vi "Update Controller State.vi"(8 "error in (no error)":errorcluster, 11 "Elevator Controller in":refnum<class "Elevator Controller.lvclass">) -> (0 "error out":errorcluster, 3 "Elevator Controller out":refnum<class "Elevator Controller.lvclass">)   [LabVIEW 2019, in "Elevator Controller.lvlib" / "Elevator Controller.lvclass"]
uses:
  Elevator Controller.lvclass
  C:/Program Files (x86)/National Instruments/LabVIEW 2019/vi.lib/ActorFramework/Actor/Actor.lvclass
  <vilib>/ActorFramework/Actor/Actor.lvclass/Actor.ctl
  <vilib>/ActorFramework/Message Enqueuer/Message Enqueuer.lvclass/Message Enqueuer.ctl
  Elevator Controller.lvclass/Elevator Controller.ctl
  Sim User Console Actor/Elevator Controller/Doors -Button.ctl
  Sim User Console Actor/Elevator Controller/Elevator Call -Cluster.ctl
  Sim User Console Actor/Elevator Controller/Floor Selection -Cluster.ctl
  Sim Display Console Actor/Elevator Controller/Elevator Direction.ctl
  Sim Display Console Actor/Elevator Controller/Floors -Enum.ctl
  Configuration Database Actor/Configuration Database Actor Messages/Write DB Msg/Write DB Msg.lvclass/Write DB Msg.ctl
  Sim Sensor Interface Actor/Sim Sensor Interface Actor Messages/Write Elevator Position Msg/Write Elevator Position Msg.lvclass/Write Elevator Position Msg.ctl
  Sim Display Console Actor/Sim Display Console Actor Messages/Write Door Open Msg/Write Door Open Msg.lvclass/Write Door Open Msg.ctl
  Sim Display Console Actor/Sim Display Console Actor Messages/Write Elevator Direction Msg/Write Elevator Direction Msg.lvclass/Write Elevator Direction Msg.ctl
  Sim Display Console Actor/Sim Display Console Actor Messages/Write Elevator Location Msg/Write Elevator Location Msg.lvclass/Write Elevator Location Msg.ctl
  Sim Display Console Actor/Sim Display Console Actor Messages/Write Emergency Msg/Write Emergency Msg.lvclass/Write Emergency Msg.ctl
  Sim Display Console Actor/Sim Display Console Actor Messages/Write Timing Msg/Write Timing Msg.lvclass/Write Timing Msg.ctl
  Sim User Console Actor/Sim User Console Actor Messages/Write Doors Msg/Write Doors Msg.lvclass/Write Doors Msg.ctl
  Sim User Console Actor/Sim User Console Actor Messages/Write Elevator Call Msg/Write Elevator Call Msg.lvclass/Write Elevator Call Msg.ctl
  Sim User Console Actor/Sim User Console Actor Messages/Write Emergency Msg/Write Emergency Msg.lvclass/Write Emergency Msg.ctl
  Sim User Console Actor/Sim User Console Actor Messages/Write Floor Selection Msg/Write Floor Selection Msg.lvclass/Write Floor Selection Msg.ctl
  State -Enum.ctl
  Elevator Controller Messages/Set State Msg/Set State Msg.lvclass/Set State Msg.ctl
  Sim User Console Actor/Sim User Console Actor Messages/Enable Doors Msg/Enable Doors Msg.lvclass/Enable Doors Msg.ctl
  Sim Display Console Actor/Sim Display Console Actor Messages/Enable Open Door Msg/Enable Open Door Msg.lvclass/Enable Open Door Msg.ctl
  Sim User Console Actor/Sim User Console Actor Messages/Enable all Controls Msg/Enable all Controls Msg.lvclass/Enable all Controls Msg.ctl
  <vilib>/ActorFramework/Message Enqueuer/Init from Existing Queue.vi
  <vilib>/ActorFramework/Message Enqueuer/Enqueue.vi
  Configuration Database Actor/Configuration Database Actor Messages/Write DB Msg/Write DB Msg.lvclass
  C:/Program Files (x86)/National Instruments/LabVIEW 2019/vi.lib/ActorFramework/Message/Message.lvclass
  Configuration Database Actor/Configuration Database Actor Messages/Read DB Msg/Read DB Msg.lvclass
  Sim Sensor Interface Actor/Sim Sensor Interface Actor Messages/Write Elevator Position Msg/Write Elevator Position Msg.lvclass
  Sim Display Console Actor/Sim Display Console Actor Messages/Write Door Open Msg/Write Door Open Msg.lvclass
  Sim Display Console Actor/Sim Display Console Actor Messages/Write Elevator Direction Msg/Write Elevator Direction Msg.lvclass
  Sim Display Console Actor/Sim Display Console Actor Messages/Write Elevator Location Msg/Write Elevator Location Msg.lvclass
  Sim Display Console Actor/Sim Display Console Actor Messages/Write Emergency Msg/Write Emergency Msg.lvclass
  Sim Display Console Actor/Sim Display Console Actor Messages/Write Timing Msg/Write Timing Msg.lvclass
  Sim User Console Actor/Sim User Console Actor Messages/Write Doors Msg/Write Doors Msg.lvclass
  Sim User Console Actor/Sim User Console Actor Messages/Write Elevator Call Msg/Write Elevator Call Msg.lvclass
  Sim User Console Actor/Sim User Console Actor Messages/Write Emergency Msg/Write Emergency Msg.lvclass
  Sim User Console Actor/Sim User Console Actor Messages/Write Floor Selection Msg/Write Floor Selection Msg.lvclass
  Elevator Controller Messages/Set State Msg/Set State Msg.lvclass
  Sim User Console Actor/Sim User Console Actor Messages/Enable Doors Msg/Enable Doors Msg.lvclass
  Sim Display Console Actor/Sim Display Console Actor Messages/Read Elevator Direction Msg/Read Elevator Direction Msg.lvclass
  Sim User Console Actor/Sim User Console Actor Messages/Read All Controls Msg/Read All Controls Msg.lvclass
  Elevator Controller Messages/Analysis Msg/Analysis Msg.lvclass
  Sim Display Console Actor/Sim Display Console Actor Messages/Enable Open Door Msg/Enable Open Door Msg.lvclass
  Sim User Console Actor/Sim User Console Actor Messages/Enable all Controls Msg/Enable all Controls Msg.lvclass
  <vilib>/ActorFramework/Message Priority Queue/Priority Enqueue.vi
  <vilib>/ActorFramework/Message Enqueuer/Message Enqueuer.lvclass
  <vilib>/ActorFramework/Actor/Actor.lvclass
  Sim User Console Actor/Elevator Controller/Sim User Console Actor.lvclass
  Sim Display Console Actor/Elevator Controller/Sim Display Console Actor.lvclass
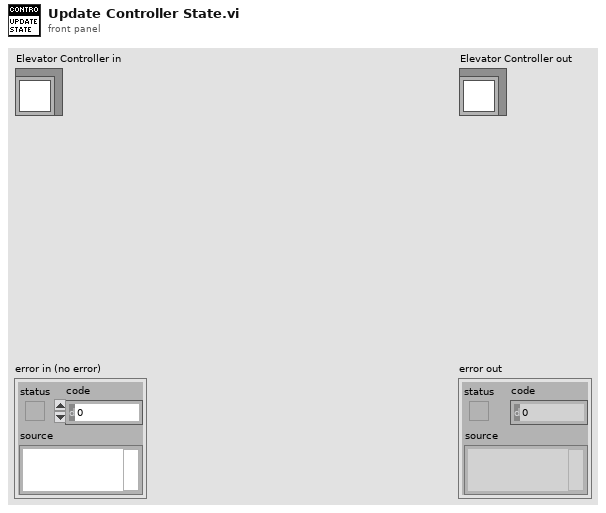
[diagram p1: front panel]
types:
  T1 = typedef "Sim Display Console Actor.lvlib/Sim Display Console Actor.lvclass/Floors -Enum.ctl" = enum16{"1st Floor", "2nd Floor", "3rd Floor", "4th Floor"}
  T2 = typedef "Sim Display Console Actor.lvlib/Sim Display Console Actor.lvclass/Elevator Direction.ctl" = cluster{"Open Door":bool, "Close Door":bool}
  T3 = typedef "Sim User Console Actor.lvlib/Sim User Console Actor.lvclass/Floor Selection -Cluster.ctl" = cluster{"4":bool, "3":bool, "2":bool, "1":bool}
  T4 = typedef "Sim User Console Actor.lvlib/Sim User Console Actor.lvclass/Elevator Call -Cluster.ctl" = cluster{"Up 3":bool, "Up 2":bool, "Up 1":bool, "Down 4":bool, "Down 3":bool, "Down 2":bool}
  T5 = typedef "Sim User Console Actor.lvlib/Sim User Console Actor.lvclass/Doors -Button.ctl" = cluster{"Open Door":bool, "Close Door":bool}
  T6 = typedef "Elevator Controller.lvlib/Elevator Controller.lvclass/State -Enum.ctl" = enum16{"Initial", "Wait for First Request", "Start and Move", "Analysis", "Continue Travel", "Stop at Floor", "Open and Close Door Sequence", "No request Remaining", "Emergency Call", "Terminate Process"}
  T7 = enum8{"Enabled", "Disabled", "Disabled and Grayed Out"}
  T8 = typedef "Configuration Database Actor.lvlib/Configuration Database Actor.lvclass/Record Data -Cluster.ctl" = cluster{"Door Open":dbl, "Door Close":dbl, "Travel Time":dbl, "Inactivity Time":dbl}
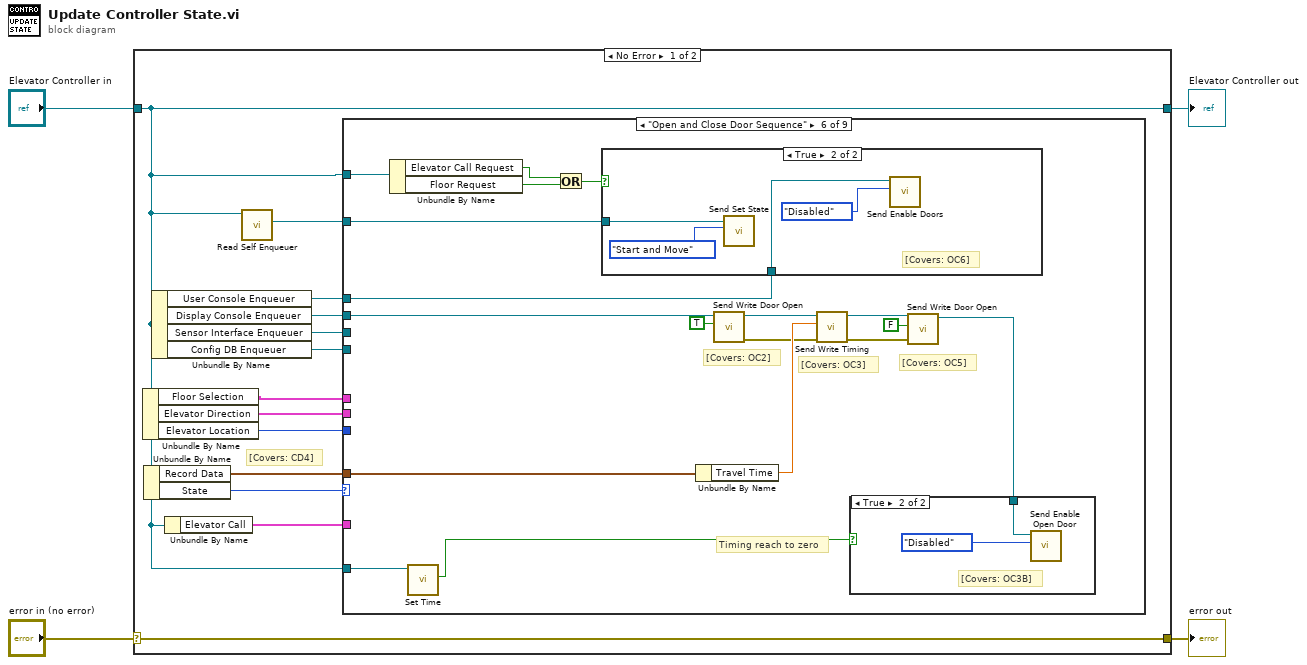
[diagram p0: block diagram]
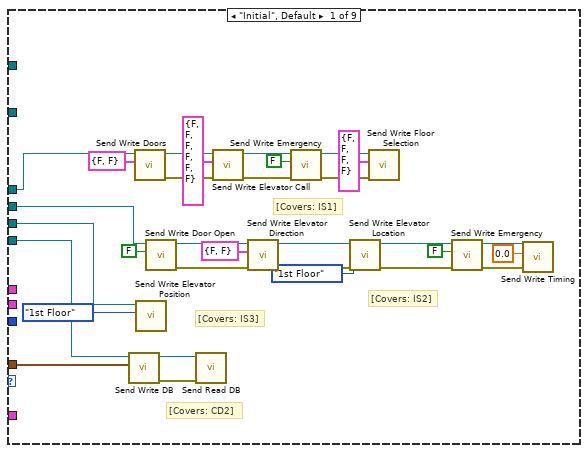
[diagram p2: hidden frame]
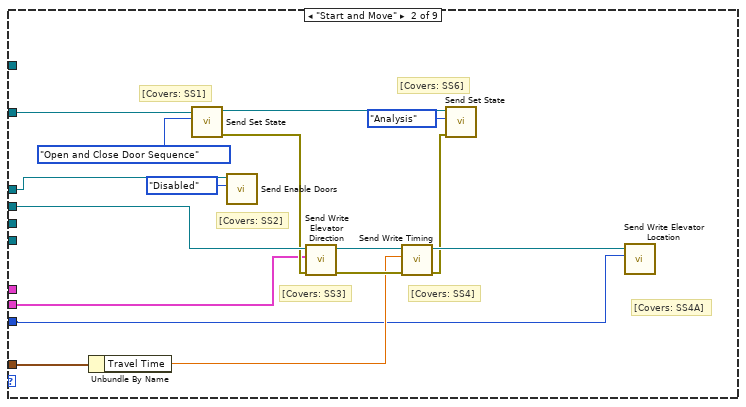
[diagram p3: hidden frame]
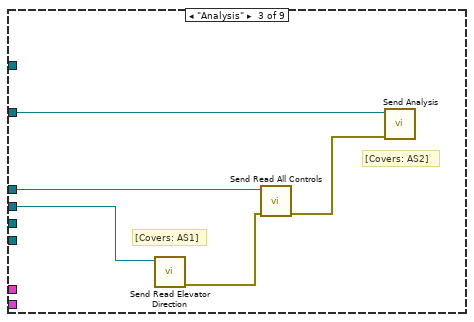
[diagram p4: hidden frame]
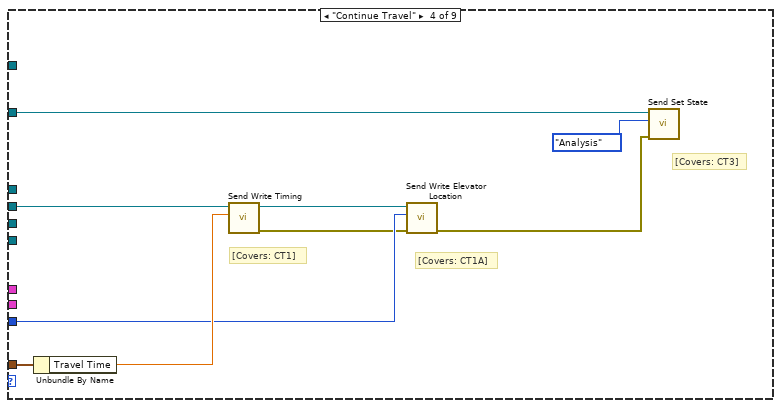
[diagram p5: hidden frame]
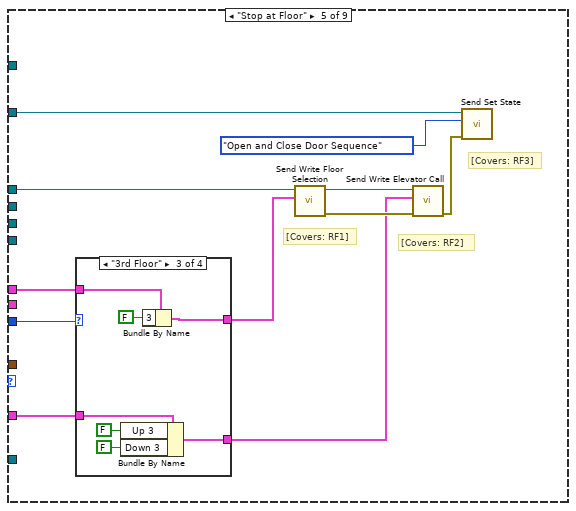
[diagram p6: hidden frame]
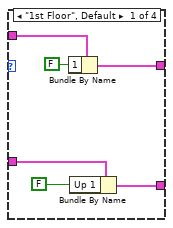
[diagram p7: hidden frame]
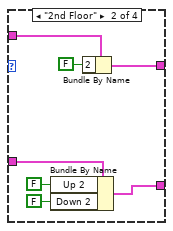
[diagram p8: hidden frame]
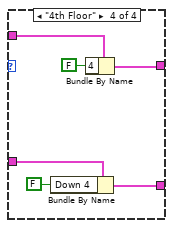
[diagram p9: hidden frame]
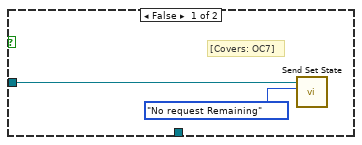
[diagram p11: hidden frame]
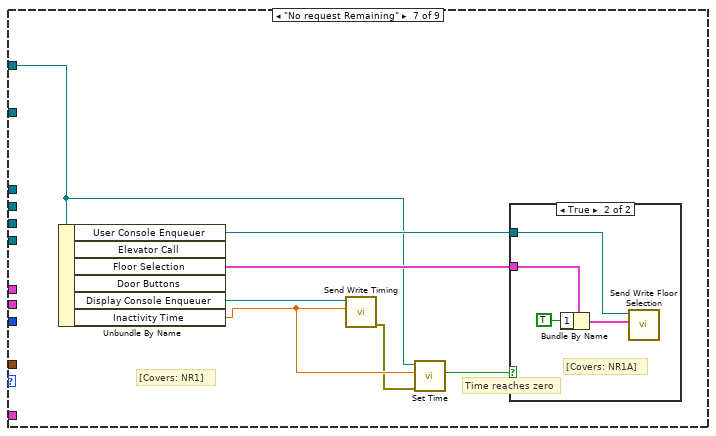
[diagram p12: hidden frame]
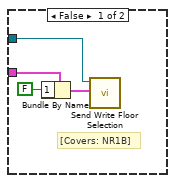
[diagram p13: hidden frame]
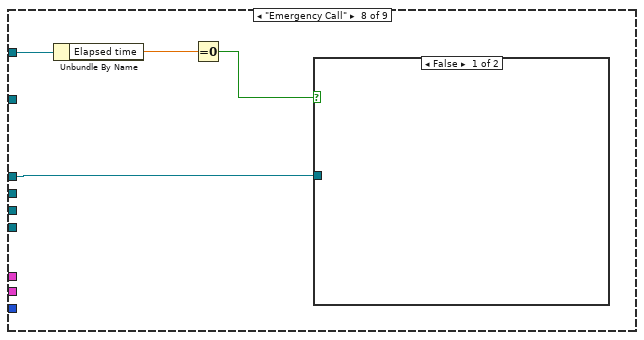
[diagram p14: hidden frame]
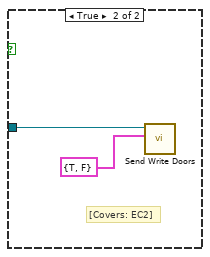
[diagram p15: hidden frame]
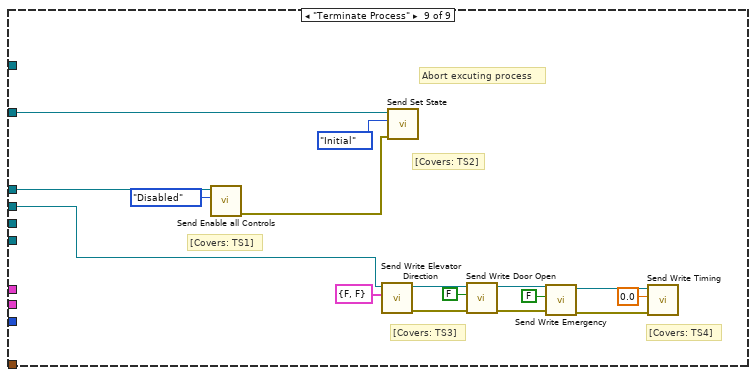
[diagram p16: hidden frame]
diagram:
  n1 = case shown="No Error" "error in (no error)" {
    selector: "error in (no error)" -> [w17 w180]
    tunnel: [w17 w180] -> w3
    tunnel: [w5 w179] -> w1
    tunnel: "Elevator Controller in" -> [w5 w179]
    frame No Error {
      # "[Covers: CD4]"
      n2 = Unbundle By Name(w5) -> ("Floor Selection"=w7:T3, "Elevator Direction"=w9:T2, "Elevator Location"=w8:T1)
      n3 = Unbundle By Name(w5) -> ("Record Data"=w10:T8, "State"=w16:T6)
      n4 = Unbundle By Name(w5) -> ("User Console Enqueuer"=w15:refnum<class "Message Enqueuer.lvclass">, "Display Console Enqueuer"=w14:refnum<class "Message Enqueuer.lvclass">, "Sensor Interface Enqueuer"=w13:refnum<class "Message Enqueuer.lvclass">, "Config DB Enqueuer"=w12:refnum<class "Message Enqueuer.lvclass">)
      n5 = Unbundle By Name(w5) -> ("Elevator Call"=w6:T4)
      n6 = call <vilib>:"Read Self Enqueuer.vi"("Actor"=w5) -> ("Self Enqueuer"=w11:refnum<class "Message Enqueuer.lvclass">)  [unwired: 10 in]
      n7 = case shown="\"Open and Close Door Sequence\"" w16 {
        tunnel: w15 -> [w44 w62 w69 _ w89 w122 _ w158 w178]
        tunnel: w14 -> [w25 w60 w68 w75 _ w133 _ _ w166]
        tunnel: w13 -> [w19 _ _ _ _ _ _ _ _]
        tunnel: w12 -> [w48 _ _ _ _ _ _ _ _]
        tunnel: w11 -> [_ w64 w67 w78 w81 w120 _ _ w176]
        tunnel: w10 -> [w45 w59 _ w76 _ w130 _ _ _]
        tunnel: w9 -> [_ w49 _ _ _ _ _ _ _]
        tunnel: w5 -> [_ _ _ _ _ w125 w142 w160 _]
        tunnel: w8 -> [_ w54 _ w72 w88 _ _ _ _]
        tunnel: w7 -> [_ _ _ _ w86 _ _ _ _]
        tunnel: w6 -> [_ _ _ _ w83 _ _ _ _]
        tunnel: w5 -> [_ _ _ _ _ w119 _ _ _]
        frame "Initial", Default {
          # "[Covers: IS3]"
          # "[Covers: IS2]"
          # "[Covers: IS1]"
          # "[Covers: CD2]"
          n8 = call "Send Write DB.vi"("Record Data"=w45, "Message Enqueuer"=w48) -> ("error out"=w46:errorcluster, "Message Enqueuer out"=w47:refnum<class "Message Enqueuer.lvclass">)  [unwired: 8 in]
          n9 = call "Send Write Doors.vi"("Door Buttons"=T5 {"Open Door"=FALSE, "Close Door"=FALSE}, "Message Enqueuer"=w44) -> ("error out"=w40:errorcluster, "Message Enqueuer out"=w43:refnum<class "Message Enqueuer.lvclass">)  [unwired: 8 in]
          n10 = call "Send Write Elevator Position.vi"("Elevator Position"=Floors_-Enum."1st Floor" ("Elevator Location"), "Message Enqueuer"=w19) -> ()  [unwired: 8 in, 2 out]
          n11 = call "Send Write Door Open.vi"("Door Open"=FALSE, "Message Enqueuer"=w25) -> ("error out"=w29:errorcluster, "Message Enqueuer out"=w33:refnum<class "Message Enqueuer.lvclass">)  [unwired: 8 in]
          n12 = call "Send Read DB.vi"("error in (no error)"=w46, "Message Enqueuer"=w47) -> ()  [unwired: 8 in, 2 out]
          n13 = call "Send Write Elevator Call.vi"("error in (no error)"=w40, "Elevator Call"=T4 {"Up 3"=FALSE, "Up 2"=FALSE, "Up 1"=FALSE, "Down 4"=FALSE, "Down 3"=FALSE, "Down 2"=FALSE}, "Message Enqueuer"=w43) -> ("error out"=w39:errorcluster, "Message Enqueuer out"=w42:refnum<class "Message Enqueuer.lvclass">)  [unwired: 7 in]
          n14 = call "Send Write Elevator Direction.vi"("error in (no error)"=w29, "Elevator Direction"=T2 {"Open Door"=FALSE, "Close Door"=FALSE}, "Message Enqueuer"=w33) -> ("error out"=w28:errorcluster, "Message Enqueuer out"=w32:refnum<class "Message Enqueuer.lvclass">)  [unwired: 7 in]
          n15 = call "Send Write Emergency.vi"("error in (no error)"=w39, "Emergency"=FALSE, "Message Enqueuer"=w42) -> ("error out"=w38:errorcluster, "Message Enqueuer out"=w41:refnum<class "Message Enqueuer.lvclass">)  [unwired: 7 in]
          n16 = call "Send Write Elevator Location.vi"("error in (no error)"=w28, "Elevator Location"=Floors_-Enum."1st Floor", "Message Enqueuer"=w32) -> ("error out"=w27:errorcluster, "Message Enqueuer out"=w31:refnum<class "Message Enqueuer.lvclass">)  [unwired: 7 in]
          n17 = call "Send Write Floor Selection.vi"("error in (no error)"=w38, "Floor Selection"=T3 {"4"=FALSE, "3"=FALSE, "2"=FALSE, "1"=FALSE}, "Message Enqueuer"=w41) -> ()  [unwired: 7 in, 2 out]
          n18 = call "Send Write Emergency.vi"("error in (no error)"=w27, "Emergency"=FALSE, "Message Enqueuer"=w31) -> ("error out"=w26:errorcluster, "Message Enqueuer out"=w30:refnum<class "Message Enqueuer.lvclass">)  [unwired: 7 in]
          n19 = call "Send Write Timing.vi"("error in (no error)"=w26, "timing"=0.0, "Message Enqueuer"=w30) -> ()  [unwired: 7 in, 2 out]
        }
        frame "Start and Move" {
          # "[Covers: SS4A]"
          # "[Covers: SS6]"
          # "[Covers: SS4]"
          # "[Covers: SS3]"
          # "[Covers: SS2]"
          # "[Covers: SS1]"
          n20 = Unbundle By Name(w59) -> ("Travel Time"=w56:dbl)
          n21 = call "Send Set State.vi"("State"=State_-Enum."Open and Close Door Sequence", "Message Enqueuer"=w64) -> ("error out"=w52:errorcluster, "Message Enqueuer out"=w51:refnum<class "Message Enqueuer.lvclass">)  [unwired: 8 in]
          n22 = call "Send Enable Doors.vi"("Disabled"=T7."Disabled", "Message Enqueuer"=w62) -> ()  [unwired: 8 in, 2 out]
          n23 = call "Send Write Elevator Direction.vi"("error in (no error)"=w52, "Elevator Direction"=w49, "Message Enqueuer"=w60) -> ("error out"=w57:errorcluster, "Message Enqueuer out"=w58:refnum<class "Message Enqueuer.lvclass">)  [unwired: 7 in]
          n24 = call "Send Write Timing.vi"("error in (no error)"=w57, "timing"=w56, "Message Enqueuer"=w58) -> ("error out"=w53:errorcluster, "Message Enqueuer out"=w55:refnum<class "Message Enqueuer.lvclass">)  [unwired: 7 in]
          n25 = call "Send Set State.vi"("error in (no error)"=w53, "State"=State_-Enum."Analysis", "Message Enqueuer"=w51) -> ()  [unwired: 7 in, 2 out]
          n26 = call "Send Write Elevator Location.vi"("Elevator Location"=w54, "Message Enqueuer"=w55) -> ()  [unwired: 8 in, 2 out]
        }
        frame "Analysis" {
          # "[Covers: AS2]"
          # "[Covers: AS1]"
          n27 = call "Send Read Elevator Direction.vi"("Message Enqueuer"=w68) -> ("error out"=w66:errorcluster)  [unwired: 9 in, 1 out]
          n28 = call "Send Read All Controls.vi"("error in (no error)"=w66, "Message Enqueuer"=w69) -> ("error out"=w65:errorcluster)  [unwired: 8 in, 1 out]
          n29 = call "Send Analysis.vi"("error in (no error)"=w65, "Message Enqueuer"=w67) -> ()  [unwired: 8 in, 2 out]
        }
        frame "Continue Travel" {
          # "[Covers: CT1A]"
          # "[Covers: CT1]"
          # "[Covers: CT3]"
          n30 = Unbundle By Name(w76) -> ("Travel Time"=w74:dbl)
          n31 = call "Send Write Timing.vi"("timing"=w74, "Message Enqueuer"=w75) -> ("error out"=w71:errorcluster, "Message Enqueuer out"=w73:refnum<class "Message Enqueuer.lvclass">)  [unwired: 8 in]
          n32 = call "Send Write Elevator Location.vi"("error in (no error)"=w71, "Elevator Location"=w72, "Message Enqueuer"=w73) -> ("error out"=w70:errorcluster)  [unwired: 7 in, 1 out]
          n33 = call "Send Set State.vi"("error in (no error)"=w70, "State"=State_-Enum."Analysis", "Message Enqueuer"=w78) -> ()  [unwired: 7 in, 2 out]
        }
        frame "Stop at Floor" {
          # "[Covers: RF3]"
          # "[Covers: RF2]"
          # "[Covers: RF1]"
          n34 = case shown="\"3rd Floor\"" w88 {
            tunnel: w86 -> [w95 w100 w107 w113]
            tunnel: [w93 w101 w108 w114] -> w87
            tunnel: w83 -> [w91 w99 w106 w112]
            tunnel: [w90 w98 w105 w110] -> w82
            frame "1st Floor", Default {
              n35 = Bundle By Name(cluster=w95, "1"=FALSE) -> (w93:T3)
              n36 = Bundle By Name(cluster=w91, "Up 1"=FALSE ("Down 4")) -> (w90:T4)
            }
            frame "2nd Floor" {
              n37 = Bundle By Name(cluster=w99, "Up 2"=FALSE, "Down 2"=FALSE) -> (w98:T4)
              n38 = Bundle By Name(cluster=w100, "2"=FALSE ("1")) -> (w101:T3)
            }
            frame "3rd Floor" {
              n39 = Bundle By Name(cluster=w106, "Up 3"=FALSE, "Down 3"=FALSE) -> (w105:T4)
              n40 = Bundle By Name(cluster=w107, "3"=FALSE ("1")) -> (w108:T3)
            }
            frame "4th Floor" {
              n41 = Bundle By Name(cluster=w112, "Down 4"=FALSE) -> (w110:T4)
              n42 = Bundle By Name(cluster=w113, "4"=FALSE ("1")) -> (w114:T3)
            }
          }
          n43 = call "Send Write Floor Selection.vi"("Floor Selection"=w87, "Message Enqueuer"=w89) -> ("error out"=w84:errorcluster, "Message Enqueuer out"=w85:refnum<class "Message Enqueuer.lvclass">)  [unwired: 8 in]
          n44 = call "Send Write Elevator Call.vi"("error in (no error)"=w84, "Elevator Call"=w82, "Message Enqueuer"=w85) -> ("error out"=w80:errorcluster)  [unwired: 7 in, 1 out]
          n45 = call "Send Set State.vi"("error in (no error)"=w80, "State"=State_-Enum."Open and Close Door Sequence", "Message Enqueuer"=w81) -> ()  [unwired: 7 in, 2 out]
        }
        frame "Open and Close Door Sequence" {
          # "Timing reach to zero"
          # "[Covers: OC5]"
          # "[Covers: OC3]"
          # "[Covers: OC2]"
          n46 = Unbundle By Name(w125) -> ("Elevator Call Request"=w124:bool, "Floor Request"=w123:bool)
          n47 = call "Set Time.vi"("Elevator Controller in"=w119) -> ("Done"=w117:bool)  [unwired: 8 in, 2 out]
          n48 = Or(x=w124, y=w123) -> (x .or. y?=w121:bool)
          n49 = case shown="True" w121 {
            tunnel: w122 -> [_ w140]
            tunnel: w120 -> [w136 w139]
            frame False {
              # "[Covers: OC7]"
              n50 = call "Send Set State.vi"("State"=State_-Enum."No request Remaining", "Message Enqueuer"=w136) -> ()  [unwired: 8 in, 2 out]
            }
            frame True {
              # "[Covers: OC6]"
              n51 = call "Send Set State.vi"("State"=State_-Enum."Start and Move", "Message Enqueuer"=w139) -> ()  [unwired: 8 in, 2 out]
              n52 = call "Send Enable Doors.vi"("Disabled"=T7."Disabled", "Message Enqueuer"=w140) -> ()  [unwired: 8 in, 2 out]
            }
          }
          n53 = Unbundle By Name(w130) -> ("Travel Time"=w131:dbl)
          n54 = call "Send Write Door Open.vi"("Door Open"=TRUE, "Message Enqueuer"=w133) -> ("error out"=w118:errorcluster, "Message Enqueuer out"=w129:refnum<class "Message Enqueuer.lvclass">)  [unwired: 8 in]
          n55 = call "Send Write Timing.vi"("error in (no error)"=w118, "timing"=w131, "Message Enqueuer"=w129) -> ("error out"=w127:errorcluster, "Message Enqueuer out"=w128:refnum<class "Message Enqueuer.lvclass">)  [unwired: 7 in]
          n56 = call "Send Write Door Open.vi"("error in (no error)"=w127, "Door Open"=FALSE, "Message Enqueuer"=w128) -> ("Message Enqueuer out"=w116:refnum<class "Message Enqueuer.lvclass">)  [unwired: 7 in, 1 out]
          n57 = case shown="True" w117 {
            tunnel: w116 -> [_ w135]
            frame False {
            }
            frame True {
              # "[Covers: OC3B]"
              n58 = call "Send Enable Open Door.vi"("Disabled"=T7."Disabled", "Message Enqueuer"=w135) -> ()  [unwired: 8 in, 2 out]
            }
          }
        }
        frame "No request Remaining" {
          # "Time reaches zero"
          # "[Covers: NR1]"
          n59 = Unbundle By Name(w142) -> ("User Console Enqueuer"=w146:refnum<class "Message Enqueuer.lvclass">, "Floor Selection"=w143:T3, "Display Console Enqueuer"=w148:refnum<class "Message Enqueuer.lvclass">, "Inactivity Time"=w147:dbl)  [unwired: 2 out]
          n60 = call "Send Write Timing.vi"("timing"=w147, "Message Enqueuer"=w148) -> ("error out"=w145:errorcluster)  [unwired: 8 in, 1 out]
          n61 = call "Set Time.vi"("error in (no error)"=w145, "Target time"=w147, "Elevator Controller in"=w142) -> ("Done"=w144:bool)  [unwired: 6 in, 2 out]
          n62 = case shown="True" w144 {
            tunnel: w146 -> [w152 w156]
            tunnel: w143 -> [w151 w155]
            frame False {
              # "[Covers: NR1B]"
              n63 = Bundle By Name(cluster=w151, "1"=FALSE) -> (w149:T3)
              n64 = call "Send Write Floor Selection.vi"("Floor Selection"=w149, "Message Enqueuer"=w152) -> ()  [unwired: 8 in, 2 out]
            }
            frame True {
              # "[Covers: NR1A]"
              n65 = Bundle By Name(cluster=w155, "1"=TRUE) -> (w154:T3)
              n66 = call "Send Write Floor Selection.vi"("Floor Selection"=w154, "Message Enqueuer"=w156) -> ()  [unwired: 8 in, 2 out]
            }
          }
        }
        frame "Emergency Call" {
          n67 = Unbundle By Name(w160) -> ("Elapsed time"=w159:dbl)
          n68 = Equal To 0?(x=w159) -> (x = 0?=w157:bool)
          n69 = case shown="False" w157 {
            tunnel: w158 -> [_ w162]
            frame False {
            }
            frame True {
              # "[Covers: EC2]"
              n70 = call "Send Write Doors.vi"("Door Buttons"=T5 {"Open Door"=TRUE, "Close Door"=FALSE}, "Message Enqueuer"=w162) -> ()  [unwired: 8 in, 2 out]
            }
          }
        }
        frame "Terminate Process" {
          # "[Covers: TS4]"
          # "[Covers: TS3]"
          # "[Covers: TS2]"
          # "Abort excuting process"
          # "[Covers: TS1]"
          n71 = call "Send Enable all Controls.vi"("Disabled"=T7."Disabled", "Message Enqueuer"=w178) -> ("error out"=w174:errorcluster)  [unwired: 8 in, 1 out]
          n72 = call "Send Write Elevator Direction.vi"("Elevator Direction"=T2 {"Open Door"=FALSE, "Close Door"=FALSE}, "Message Enqueuer"=w166) -> ("error out"=w168:errorcluster, "Message Enqueuer out"=w167:refnum<class "Message Enqueuer.lvclass">)  [unwired: 8 in]
          n73 = call "Send Set State.vi"("error in (no error)"=w174, "State"=State_-Enum."Initial", "Message Enqueuer"=w176) -> ()  [unwired: 7 in, 2 out]
          n74 = call "Send Write Door Open.vi"("error in (no error)"=w168, "Door Open"=FALSE, "Message Enqueuer"=w167) -> ("error out"=w173:errorcluster, "Message Enqueuer out"=w172:refnum<class "Message Enqueuer.lvclass">)  [unwired: 7 in]
          n75 = call "Send Write Emergency.vi"("error in (no error)"=w173, "Emergency"=FALSE, "Message Enqueuer"=w172) -> ("error out"=w164:errorcluster, "Message Enqueuer out"=w165:refnum<class "Message Enqueuer.lvclass">)  [unwired: 7 in]
          n76 = call "Send Write Timing.vi"("error in (no error)"=w164, "timing"=0.0, "Message Enqueuer"=w165) -> ()  [unwired: 7 in, 2 out]
        }
      }
    }
    frame Error {
    }
  }
  "error out" <- w3
  "Elevator Controller out" <- w1
